vi "Configure PWM.vi"(5 "Purpose (\"PWM\")":string="PWM", 7 "GPIO #":T1=-1, 8 "error in (no error)":errorcluster, 9 "Phase-Correct (F)":bool, 10 "Enable (F)":bool, 11 "Session in":refnum<class "Session.lvclass">) -> (0 "error out":errorcluster, 3 "Session out":refnum<class "Session.lvclass">)   [LabVIEW 2024, in "CTI.lvlib" / "Session.lvclass"]
doc: "PWM is useful for actions such as brightness controlling LEDs, controlling RC servos, and acting like an analog output by varying the duty cycle."
uses:
  Session.lvclass
  GPIO Number.ctl
  Session.lvclass/Session.ctl
  6d685646-5fc2-4306-aced-85eeb5eb8c91.vi
  Is Full Errors.vi
  Check Errors.vi
  CTI.lvlib
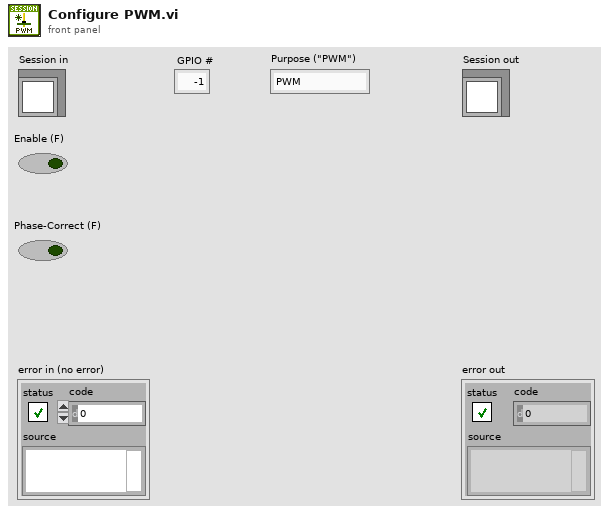
[diagram p1: front panel]
types:
  T1 = typedef "CTI.lvlib/GPIO Number.ctl" = i8
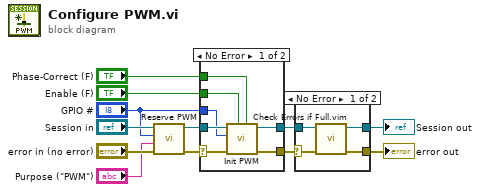
[diagram p0: block diagram]
diagram:
  n1 = call "Reserve PWM.vi"("error in (no error)"="error in (no error)", "Purpose"="Purpose (\"PWM\")", "GPIO #"="GPIO #", "Session in"="Session in") -> ("error out"=w11:errorcluster, "Session out"=w8:refnum<class "Session.lvclass">)  [unwired: 6 in]
  n2 = case shown="No Error" w11 {
    selector: w11 -> [w19 w20]
    tunnel: [w18 w20] -> w7
    tunnel: w8 -> [w17 w21]
    tunnel: [w16 w21] -> w6
    tunnel: "Enable (F)" -> [w15 _]
    tunnel: "Phase-Correct (F)" -> [w14 _]
    tunnel: "GPIO #" -> [w13 _]
    frame No Error {
      n3 = call "Init PWM.vi"("Phase-Correct (F)"=w14, "Enable (T)"=w15, "error in (no error)"=w19, "GPIO #"=w13, "Session in"=w17) -> ("error out"=w18:errorcluster, "Session out"=w16:refnum<class "Session.lvclass">)  [unwired: 5 in]
    }
    frame Error {
    }
  }
  n4 = case shown="No Error" w7 {
    selector: w7 -> [w22 w26]
    tunnel: w6 -> [w23 w27]
    tunnel: [w25 w26] -> w5
    tunnel: [w24 w27] -> w4
    frame No Error {
      n5 = call "Check Errors if Full.vim"("error in (no error)"=w22, "Session in"=w23) -> ("error out"=w25:errorcluster, "Session out"=w24:refnum<class "Session.lvclass">)  [unwired: 8 in]
    }
    frame Error {
    }
  }
  "error out" <- w5
  "Session out" <- w4
